vi "Plot Impulses.vi"(8 "error in (no error)":errorcluster, 10 "Graph Manager":refnum<class "Graph Manager.lvclass">, 11 "Impulse Manager in":refnum<class "Impulse Manager.lvclass">) -> (0 "error out":errorcluster, 2 "Graph Manager out":refnum<class "Graph Manager.lvclass">, 3 "Impulse Manager out":refnum<class "Impulse Manager.lvclass">)   [LabVIEW 2016, in "Impulse Manager.lvclass"]
uses:
  Impulse Manager.lvclass
  Graph Manager/Graph Manager.lvclass
  Impulse Manager.lvclass/Impulse Manager.ctl
  Desaccade Manipulator/Desaccade Manipulator.lvclass
  Impulse Data/Impulse Data.lvclass
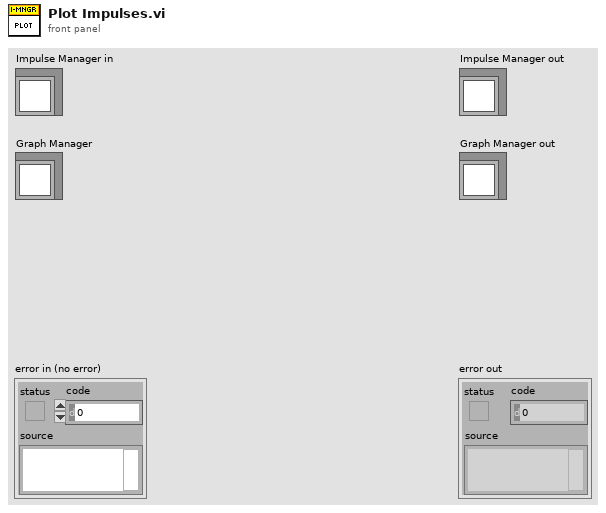
[diagram p1: front panel]
types:
  T1 = typedef "Impulse Data.lvclass/Instance handle.ctl" = refnum<data-value>
  T2 = typedef "core.lvlib/TD_Impulse Parameter.ctl" = cluster{"Color":u32, "Visible":bool, "Channel":u16, "Invert":bool, "Desaccade":bool, "Offset":dbl, "Gain":dbl}[]
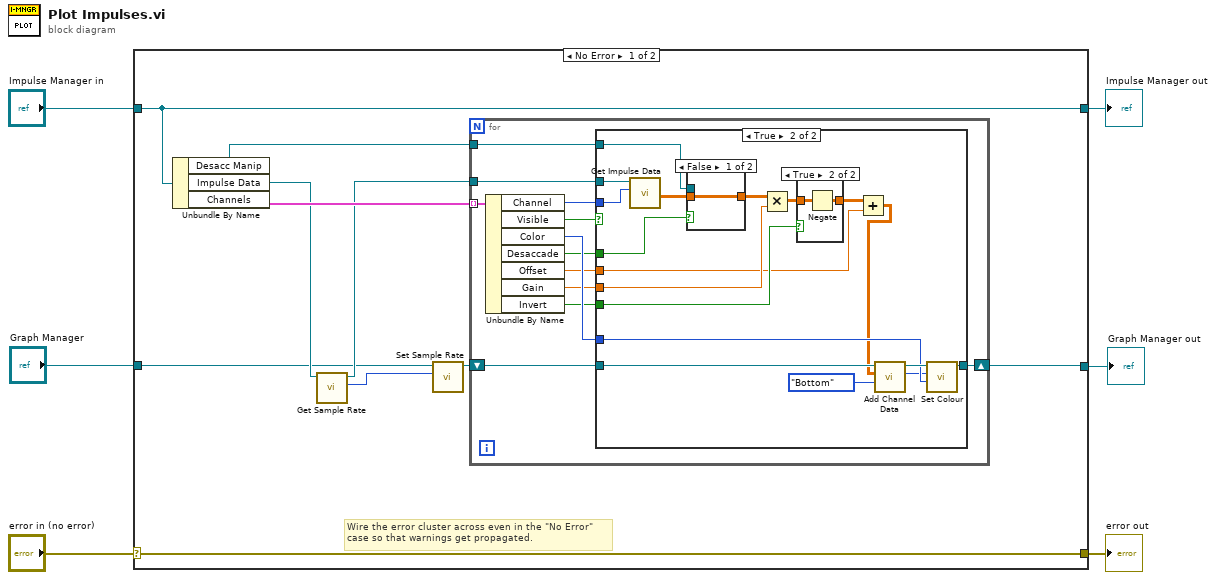
[diagram p0: block diagram]
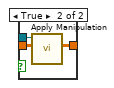
[diagram p4: hidden frame]
diagram:
  n1 = case shown="No Error" "error in (no error)" {
    selector: "error in (no error)" -> [w16 w57]
    tunnel: [w16 w57] -> w5
    tunnel: [w15 w56] -> w3
    tunnel: "Impulse Manager in" -> [w15 w56]
    tunnel: "Graph Manager" -> [w8 w55]
    tunnel: [w9 w55] -> w1
    frame No Error {
      # "Wire the error cluster across even in the \"No Error\"\ncase so that warnings get propagated."
      n2 = Unbundle By Name(w15) -> ("Desacc Manip"=w7:refnum<class "Desaccade Manipulator.lvclass">, "Impulse Data"=w11:T1, "Channels"=w14:T2)
      n3 = call "Get Sample Rate.vi"("Reference in"=w11) -> ("Sample Rate"=w10:i32, "Reference out"=w12:T1)  [unwired: 8 in, 1 out]
      n4 = call-dynamic "Set Sample Rate.vi"("Sample Rate"=w10, "Graph Manager in"=w8) -> ("Graph Manager out"=w13:refnum<class "Graph Manager.lvclass">)  [unwired: 8 in, 1 out]
      n5 = for {
        tunnel: w12 -> [w26]
        tunnel: w14 -> [w28] mode=indexing
        shift-right: [w24] -> w9
        shift-left: w13 -> [w27]
        tunnel: w7 -> [w21]
        n6 = Unbundle By Name(w28) -> ("Channel"=w25:u16, "Visible"=w22:bool, "Color"=w23:u32, "Desaccade"=w20:bool, "Offset"=w19:dbl, "Gain"=w18:dbl, "Invert"=w17:bool)
        n7 = case shown="True" w22 {
          tunnel: w27 -> [w29 w47]
          tunnel: w26 -> [_ w46]
          tunnel: w25 -> [_ w44]
          tunnel: [w29 w43] -> w24
          tunnel: w23 -> [_ w42]
          tunnel: w21 -> [_ w38]
          tunnel: w20 -> [_ w37]
          tunnel: w19 -> [_ w31]
          tunnel: w18 -> [_ w36]
          tunnel: w17 -> [_ w35]
          frame False {
          }
          frame True {
            n8 = call "Get Impulse Data.vi"("Channel"=w44, "Reference in"=w46) -> ("Impulses out"=w39:dbl[][])  [unwired: 8 in, 1 out]
            n9 = case shown="False" w37 {
              tunnel: w39 -> [w51 w54]
              tunnel: [w51 w53] -> w33
              tunnel: w38 -> [_ w52]
              frame False {
              }
              frame True {
                n10 = call-dynamic "Apply Manipulation.vi"("Data in"=w54, "Desaccade Manipulator in"=w52) -> ("Data out"=w53:dbl[][])  [unwired: 7 in, 2 out]
              }
            }
            n11 = Multiply(x=w33, y=w36) -> (x*y=w34:dbl[][])
            n12 = case shown="True" w35 {
              tunnel: w34 -> [w48 w50]
              tunnel: [w48 w49] -> w32
              frame False {
              }
              frame True {
                n13 = Negate(x=w50) -> (-x=w49:dbl[][])
              }
            }
            n14 = Add(x=w32, y=w31) -> (x+y=w30:dbl[][])
            n15 = call-dynamic "Add Channel Data.vi"("Layer"=enum16{"Top", "Bottom"}."Bottom", "Channel Data"=w30, "Graph Manager in"=w47) -> ("Channel ID"=w41:i32, "Graph Manager out"=w45:refnum<class "Graph Manager.lvclass">)  [unwired: 6 in, 1 out]
            n16 = call-dynamic "Set Colour.vi"("Color Box"=w42, "Channel in"=w41, "Graph Manager in"=w45) -> ("Graph Manager out"=w43:refnum<class "Graph Manager.lvclass">)  [unwired: 6 in, 2 out]
          }
        }
      }
    }
    frame Error {
    }
  }
  "error out" <- w5
  "Impulse Manager out" <- w3
  "Graph Manager out" <- w1
